vi "Save Controls.vi"(8 "Parent Label":string, 9 "Parent Class":string, 10 "Controls[]":refnum<vi>[](array[refnum]), 11 "Ref Config File In":T1) -> (3 "Ref Config File Out":T1)   [LabVIEW 2009]
uses:
  <vilib>/Utility/config.llb/Config Data RefNum.ctl
  <vilib>/Utility/config.llb/Write Key (Double).vi
  <vilib>/Utility/config.llb/Write Key (Boolean).vi
  <vilib>/Utility/config.llb/Write Key (String).vi
  <vilib>/Utility/config.llb/Write Key (Path).vi
  <vilib>/Utility/config.llb/Write Key (I32).vi
  <vilib>/Utility/config.llb/NI_LVConfig.lvlib
panel:
  # "Guillaume Plateau - Dec. 9, 2009\nyguig2@yahoo.fr - Version 3.0"
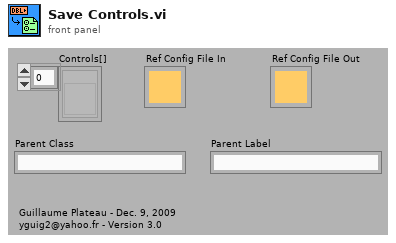
[diagram p1: front panel]
types:
  T1 = typedef "NI_LVConfig.lvlib/Config Data RefNum.ctl" = refnum<k1>
  T2 = enum16{"fractional", "engineering", "exponential"}
  T3 = typedef "LVCursorListTypeDef.ctl" = cluster{"Name":string, "Color":u32, "Style":u8, "Point Style":u8, "Name Visible":bool, "Allow Drag":bool, "Cursor Mode":u32, "Plot":i32, "Index":i32, "Position":cluster{"X":dbl, "Y":dbl}, "X Scale":u32, "Y Scale":u32, "Watch Plots":i32[], "Watch All Plots":bool, "Plot Area":i32, "Label Offset":cluster{"X":dbl, "Y":dbl}}[]
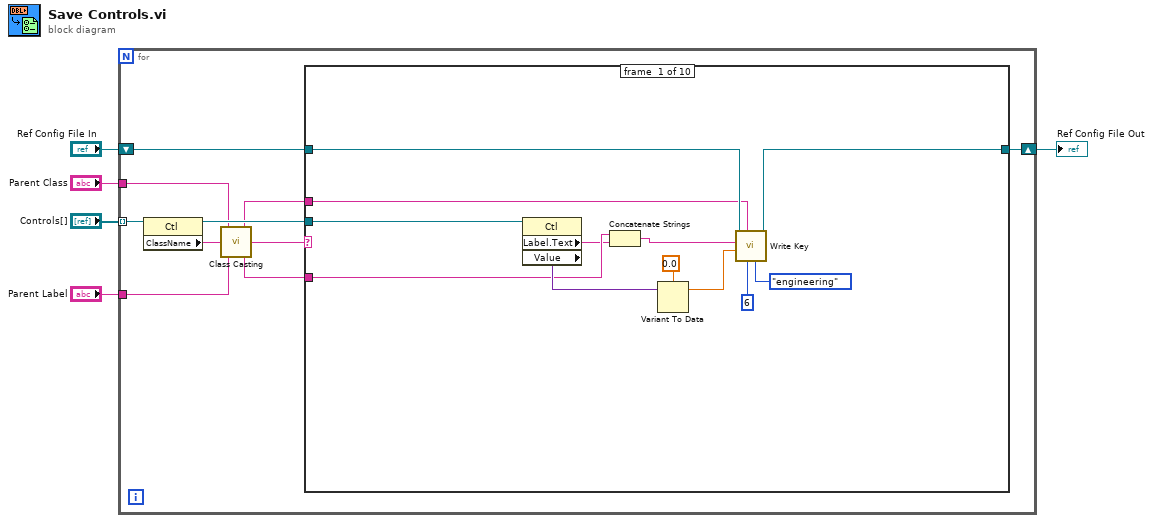
[diagram p0: block diagram]
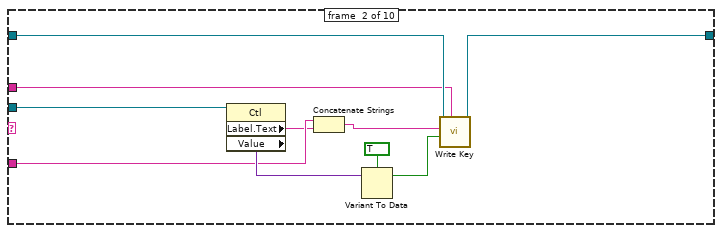
[diagram p2: hidden frame]
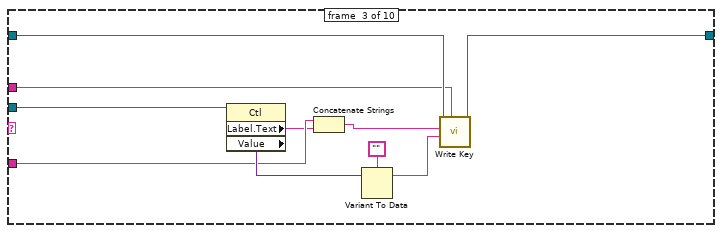
[diagram p3: hidden frame]
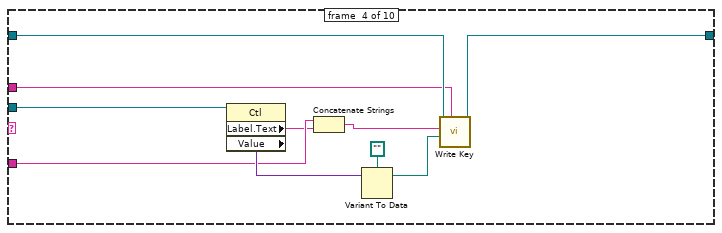
[diagram p4: hidden frame]
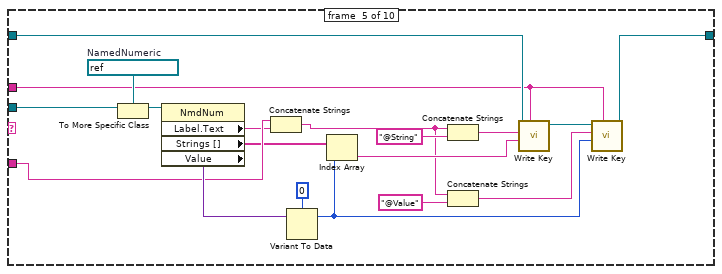
[diagram p5: hidden frame]
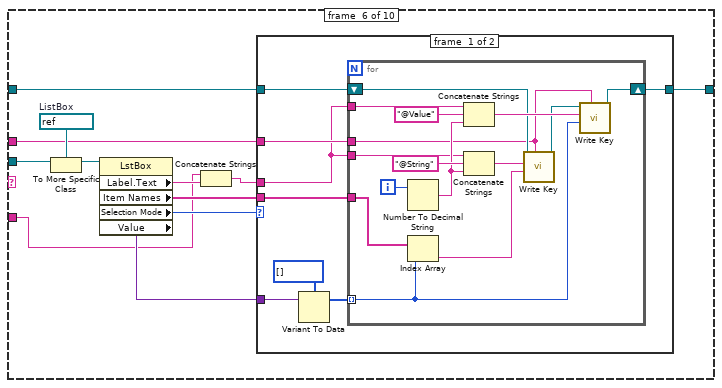
[diagram p6: hidden frame]
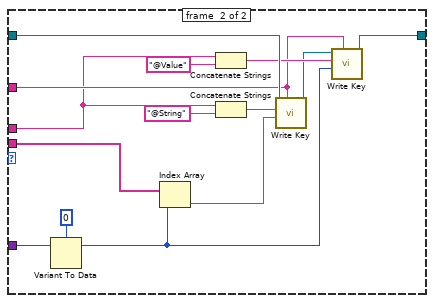
[diagram p7: hidden frame]
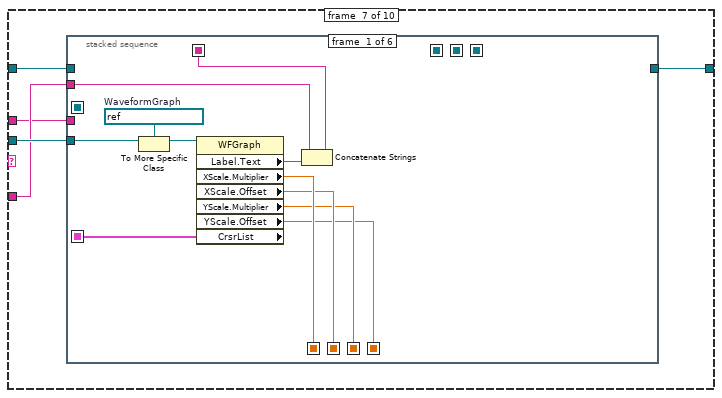
[diagram p8: hidden frame]
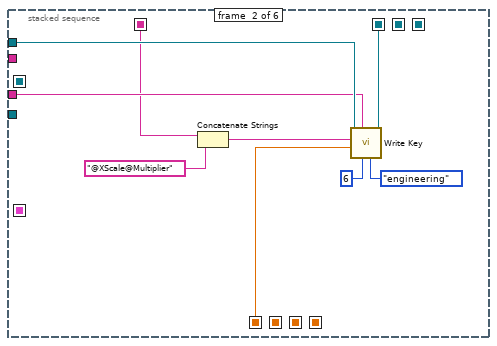
[diagram p9: hidden frame]
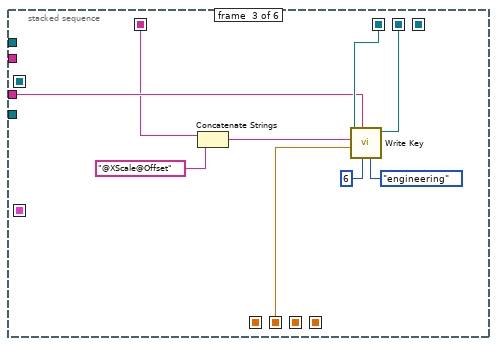
[diagram p10: hidden frame]
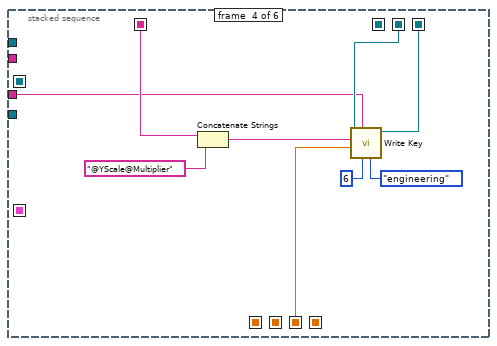
[diagram p11: hidden frame]
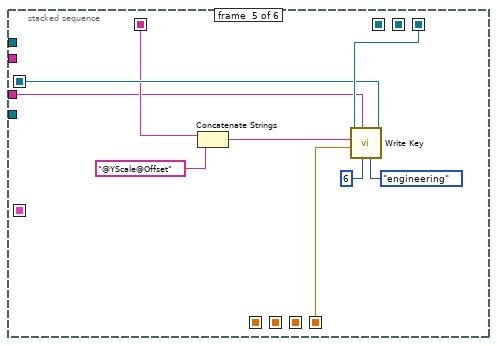
[diagram p12: hidden frame]
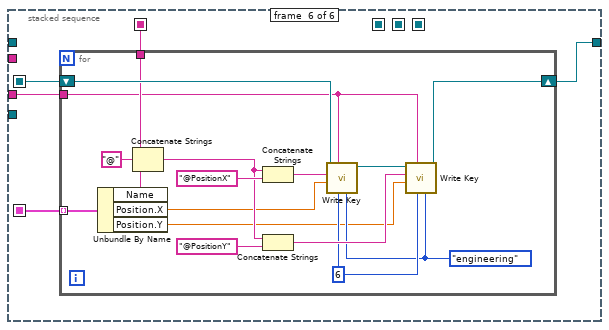
[diagram p13: hidden frame]
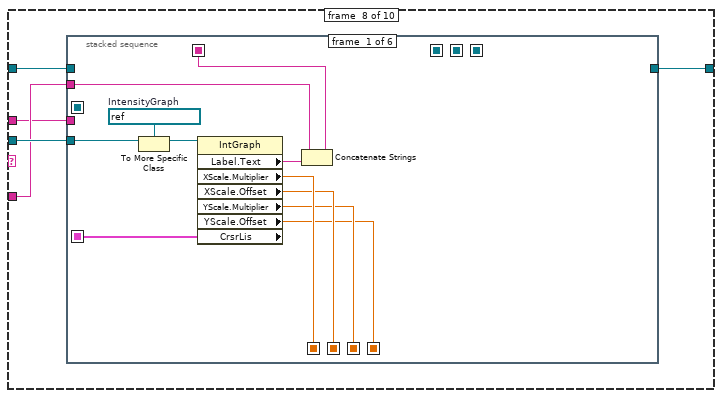
[diagram p14: hidden frame]
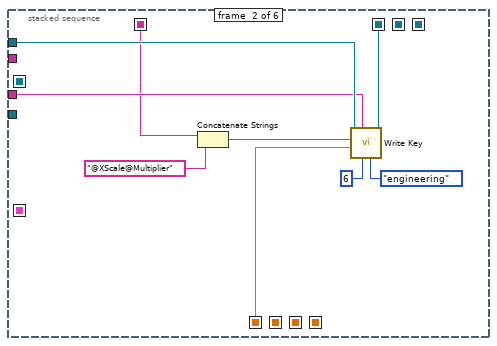
[diagram p15: hidden frame]
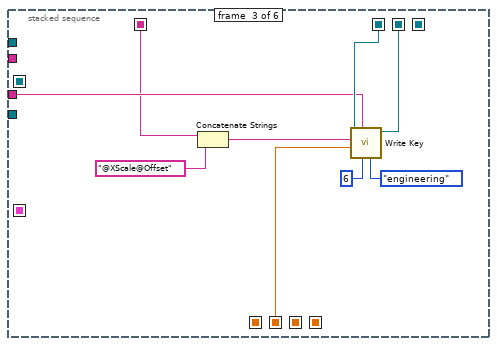
[diagram p16: hidden frame]
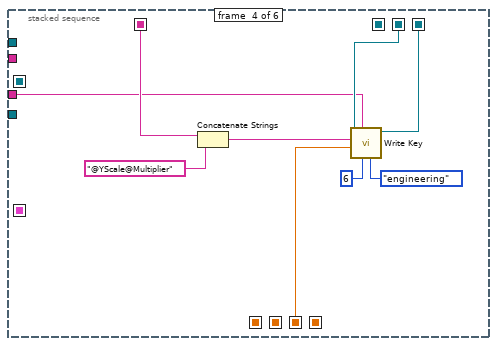
[diagram p17: hidden frame]
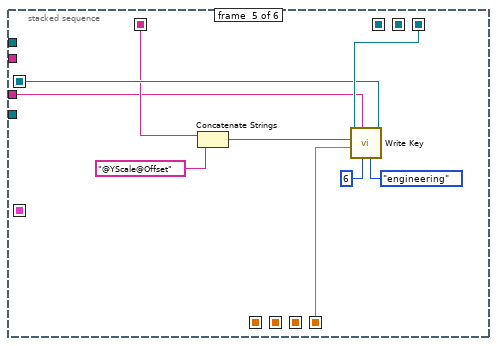
[diagram p18: hidden frame]
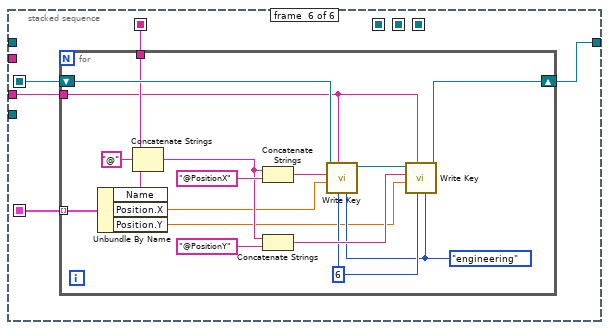
[diagram p19: hidden frame]
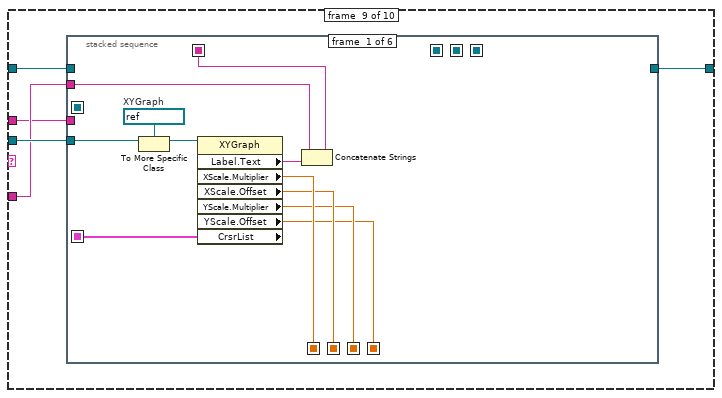
[diagram p20: hidden frame]
diagram:
  n1 = for {
    tunnel: "Controls[]" -> [w12] mode=indexing
    shift-right: [w13] -> w5
    shift-left: "Ref Config File In" -> [w14]
    tunnel: "Parent Class" -> [w7]
    tunnel: "Parent Label" -> [w11]
    n2 = property class="Ctl"(reference=w12) -> (reference out=w9:refnum<vi>, "ClassName"=w8:string)  [unwired: 1 in, 1 out]
    n3 = call "Class Casting.vi"("Parent Label"=w11, "Control Class"=w8, "Parent Class"=w7) -> ("Add-on Label"=w10:string, "Class"=w6:string)  [unwired: 1 out]
    n4 = case shown="\"OtherClasses\", Default" w8 {
      tunnel: w9 -> [w25 w27 w45 w55 w74 w87 w129 w203 w277 _]
      tunnel: w14 -> [w23 w34 w43 w53 w67 w83 w128 w202 w276 w347]
      tunnel: [w20 w32 w41 w52 w75 w80 w127 w201 w275 w347] -> w13
      tunnel: w10 -> [w19 w30 w39 w49 w61 w77 w126 w200 w274 _]
      tunnel: w6 -> [w16 w28 w37 w47 w57 w76 w125 w199 w273 _]
      frame #0 {
        n5 = property class="Ctl"(reference=w25) -> ("Label.Text"=w17:string, "Value"=w24:variant)  [unwired: 1 in, 2 out]
        n6 = Concatenate Strings(w19, w17) -> (w18:string)
        n7 = Variant To Data(Variant=w24, type=0.0) -> (data=w15:dbl)  [unwired: 1 in, 1 out]
        n8 = call-poly <vilib>:"Write Key.vi"("format (fractional)"=T2."engineering", "precision (6)"=i16 6, "section"=w16, "value"=w15, "key"=w18, "refnum"=w23) -> ("refnum out"=w20:T1)  [unwired: 2 in, 3 out]
      }
      frame #1 {
        n9 = property class="Ctl"(reference=w27) -> ("Label.Text"=w29:string, "Value"=w35:variant)  [unwired: 1 in, 2 out]
        n10 = Concatenate Strings(w30, w29) -> (w31:string)
        n11 = Variant To Data(Variant=w35, type=TRUE) -> (data=w33:bool)  [unwired: 1 in, 1 out]
        n12 = call-poly <vilib>:"Write Key.vi"("section"=w28, "value"=w33, "key"=w31, "refnum"=w34) -> ("refnum out"=w32:T1)  [unwired: 3 in, 4 out]
      }
      frame #2 {
        n13 = property class="Ctl"(reference=w45) -> ("Label.Text"=w38:string, "Value"=w44:variant)  [unwired: 1 in, 2 out]
        n14 = Concatenate Strings(w39, w38) -> (w40:string)
        n15 = Variant To Data(Variant=w44, type="") -> (data=w42:string)  [unwired: 1 in, 1 out]
        n16 = call-poly <vilib>:"Write Key.vi"("section"=w37, "value"=w42, "key"=w40, "refnum"=w43) -> ("refnum out"=w41:T1)  [unwired: 3 in, 4 out]
      }
      frame #3 {
        n17 = property class="Ctl"(reference=w55) -> ("Label.Text"=w48:string, "Value"=w54:variant)  [unwired: 1 in, 2 out]
        n18 = Concatenate Strings(w49, w48) -> (w50:string)
        n19 = Variant To Data(Variant=w54, type=path "") -> (data=w51:path)  [unwired: 1 in, 1 out]
        n20 = call-poly <vilib>:"Write Key.vi"("section"=w47, "value"=w51, "key"=w50, "refnum"=w53) -> ("refnum out"=w52:T1)  [unwired: 3 in, 4 out]
      }
      frame #4 {
        w73 = refnum<vi> refnum  # NamedNumeric
        n21 = To More Specific Class(target class=w73, reference=w74) -> (specific class reference=w72:refnum<vi>)  [unwired: 1 in, 1 out]
        n22 = property class="NmdNum"(reference=w72) -> ("Label.Text"=w60:string, "Strings []"=w58:string[], "Value"=w70:variant)  [unwired: 1 in, 2 out]
        n23 = Concatenate Strings(w61, w60) -> (w59:string)
        n24 = Variant To Data(Variant=w70, type=0) -> (data=w63:i32)  [unwired: 1 in, 1 out]
        n25 = Index Array(array=w58, index=w63) -> (element=w62:string)
        n26 = Concatenate Strings(w59, "@String" ("string")) -> (w64:string)
        n27 = Concatenate Strings(w59, "@Value" ("string")) -> (w65:string)
        n28 = call-poly <vilib>:"Write Key.vi"("section"=w57, "value"=w62, "key"=w64, "refnum"=w67) -> ("refnum out"=w66:T1)  [unwired: 2 in, 5 out]
        n29 = call-poly <vilib>:"Write Key.vi"("section"=w57, "value"=w63, "key"=w65, "refnum"=w66) -> ("refnum out"=w75:T1)  [unwired: 1 in, 6 out]
      }
      frame #5 {
        w86 = refnum<vi> refnum  # ListBox
        n30 = To More Specific Class(target class=w86, reference=w87) -> (specific class reference=w85:refnum<vi>)  [unwired: 1 in, 1 out]
        n31 = property class="LstBox"(reference=w85) -> ("Label.Text"=w79:string, "Item Names"=w81:string[], "Selection Mode"=w84:i32, "Value"=w82:variant)  [unwired: 1 in, 2 out]
        n32 = Concatenate Strings(w77, w79) -> (w78:string)
        n33 = case shown="2, 3" w84 {
          tunnel: w83 -> [w94 w124]
          tunnel: w82 -> [w93 w123]
          tunnel: w81 -> [w91 w121]
          tunnel: w76 -> [w90 w113]
          tunnel: w78 -> [w89 w112]
          tunnel: [w88 w111] -> w80
          frame #0 {
            n34 = Variant To Data(Variant=w93, type=i32[] []) -> (data=w92:i32[])  [unwired: 1 in, 1 out]
            n35 = for {
              shift-right: [w102] -> w88
              shift-left: w94 -> [w103]
              tunnel: w92 -> [w100] mode=indexing
              tunnel: w91 -> [w101]
              tunnel: w90 -> [w98]
              tunnel: w89 -> [w97]
              tunnel: w89 -> [w96]
              i -> [w108]
              n36 = Number To Decimal String(number=w108) -> (decimal integer string=w105:string)  [unwired: 1 out]
              n37 = Index Array(array=w101, index=w100) -> (element=w99:string)
              n38 = Concatenate Strings(w96, "@Value" ("string"), w105) -> (w109:string)
              n39 = Concatenate Strings(w97, "@String" ("string"), w105) -> (w107:string)
              n40 = call-poly <vilib>:"Write Key.vi"("section"=w98, "value"=w99, "key"=w107, "refnum"=w103) -> ("refnum out"=w104:T1)  [unwired: 2 in, 5 out]
              n41 = call-poly <vilib>:"Write Key.vi"("section"=w98, "value"=w100, "key"=w109, "refnum"=w104) -> ("refnum out"=w102:T1)  [unwired: 1 in, 6 out]
            }
          }
          frame #1 {
            n42 = Variant To Data(Variant=w123, type=0) -> (data=w122:i32)  [unwired: 1 in, 1 out]
            n43 = Index Array(array=w121, index=w122) -> (element=w114:string)
            n44 = Concatenate Strings(w112, "@Value" ("string")) -> (w118:string)
            n45 = Concatenate Strings(w112, "@String" ("string")) -> (w117:string)
            n46 = call-poly <vilib>:"Write Key.vi"("section"=w113, "value"=w114, "key"=w117, "refnum"=w124) -> ("refnum out"=w115:T1)  [unwired: 2 in, 5 out]
            n47 = call-poly <vilib>:"Write Key.vi"("section"=w113, "value"=w122, "key"=w118, "refnum"=w115) -> ("refnum out"=w111:T1)  [unwired: 1 in, 6 out]
          }
        }
      }
      frame #6 {
        n48 = stacked-sequence {
          seq-local: [w137 _ _ _ _ _] -> [_ _ _ _ _ w181]
          seq-local: [_ _ _ _ w170 _] -> [_ _ _ _ _ w180]
          seq-local: [w136 _ _ _ _ _] -> [_ w147 _ _ _ _]
          seq-local: [w135 _ _ _ _ _] -> [_ _ w152 _ _ _]
          seq-local: [w134 _ _ _ _ _] -> [_ _ _ w161 _ _]
          seq-local: [w133 _ _ _ _ _] -> [_ _ _ _ w171 _]
          seq-local: [_ w143 _ _ _ _] -> [_ _ w154 _ _ _]
          seq-local: [_ _ w153 _ _ _] -> [_ _ _ w163 _ _]
          seq-local: [_ _ _ w162 _ _] -> [_ _ _ _ w172 _]
          seq-local: [w130 _ _ _ _ _] -> [_ w141 w150 w160 w169 w178]
          tunnel: w129 -> [w138 _ _ _ _ _]
          tunnel: w128 -> [_ w144 _ _ _ _]
          tunnel: [_ _ _ _ _ w179] -> w127
          tunnel: w125 -> [_ w142 w151 w159 w168 w177]
          tunnel: w126 -> [w131 _ _ _ _ _]
          frame #0 {
            w140 = refnum<vi> refnum  # WaveformGraph
            n49 = To More Specific Class(target class=w140, reference=w138) -> (specific class reference=w139:refnum<vi>)  [unwired: 1 in, 1 out]
            n50 = property class="WFGraph"(reference=w139) -> ("Label.Text"=w132:string, "XScale.Multiplier"=w136:dbl, "XScale.Offset"=w135:dbl, "YScale.Multiplier"=w134:dbl, "YScale.Offset"=w133:dbl, "CrsrList"=w137:T3)  [unwired: 1 in, 2 out]
            n51 = Concatenate Strings(w131, w132) -> (w130:string)
          }
          frame #1 {
            n52 = Concatenate Strings(w141, "@XScale@Multiplier" ("string")) -> (w145:string)
            n53 = call-poly <vilib>:"Write Key.vi"("format (fractional)"=T2."engineering", "precision (6)"=i16 6, "section"=w142, "value"=w147, "key"=w145, "refnum"=w144) -> ("refnum out"=w143:T1)  [unwired: 2 in, 3 out]
          }
          frame #2 {
            n54 = Concatenate Strings(w150, "@XScale@Offset" ("string")) -> (w155:string)
            n55 = call-poly <vilib>:"Write Key.vi"("format (fractional)"=T2."engineering", "precision (6)"=i16 6, "section"=w151, "value"=w152, "key"=w155, "refnum"=w154) -> ("refnum out"=w153:T1)  [unwired: 2 in, 3 out]
          }
          frame #3 {
            n56 = Concatenate Strings(w160, "@YScale@Multiplier" ("string")) -> (w164:string)
            n57 = call-poly <vilib>:"Write Key.vi"("format (fractional)"=T2."engineering", "precision (6)"=i16 6, "section"=w159, "value"=w161, "key"=w164, "refnum"=w163) -> ("refnum out"=w162:T1)  [unwired: 2 in, 3 out]
          }
          frame #4 {
            n58 = Concatenate Strings(w169, "@YScale@Offset" ("string")) -> (w173:string)
            n59 = call-poly <vilib>:"Write Key.vi"("format (fractional)"=T2."engineering", "precision (6)"=i16 6, "section"=w168, "value"=w171, "key"=w173, "refnum"=w172) -> ("refnum out"=w170:T1)  [unwired: 2 in, 3 out]
          }
          frame #5 {
            n60 = for {
              shift-right: [w186] -> w179
              shift-left: w180 -> [w187]
              tunnel: w181 -> [w198] mode=indexing
              tunnel: w178 -> [w183]
              tunnel: w177 -> [w182]
              w190 = T2."engineering" ("format (fractional)")
              w191 = i16 6 ("precision (6)")
              n61 = Unbundle By Name(w198) -> ("Name"=w196:string, "Position.X"=w185:dbl, "Position.Y"=w184:dbl)
              n62 = Concatenate Strings(w183, "@" ("string"), w196) -> (w188:string)
              n63 = Concatenate Strings(w188, "@PositionX" ("string")) -> (w193:string)
              n64 = Concatenate Strings(w188, "@PositionY" ("string")) -> (w192:string)
              n65 = call-poly <vilib>:"Write Key.vi"("format (fractional)"=w190, "precision (6)"=w191, "section"=w182, "value"=w185, "key"=w193, "refnum"=w187) -> ("refnum out"=w189:T1)  [unwired: 2 in, 3 out]
              n66 = call-poly <vilib>:"Write Key.vi"("format (fractional)"=w190, "precision (6)"=w191, "section"=w182, "value"=w184, "key"=w192, "refnum"=w189) -> ("refnum out"=w186:T1)  [unwired: 2 in, 3 out]
            }
          }
        }
      }
      frame #7 {
        n67 = stacked-sequence {
          seq-local: [w211 _ _ _ _ _] -> [_ _ _ _ _ w255]
          seq-local: [_ _ _ _ w244 _] -> [_ _ _ _ _ w254]
          seq-local: [w210 _ _ _ _ _] -> [_ w221 _ _ _ _]
          seq-local: [w209 _ _ _ _ _] -> [_ _ w226 _ _ _]
          seq-local: [w208 _ _ _ _ _] -> [_ _ _ w235 _ _]
          seq-local: [w207 _ _ _ _ _] -> [_ _ _ _ w245 _]
          seq-local: [_ w217 _ _ _ _] -> [_ _ w228 _ _ _]
          seq-local: [_ _ w227 _ _ _] -> [_ _ _ w237 _ _]
          seq-local: [_ _ _ w236 _ _] -> [_ _ _ _ w246 _]
          seq-local: [w204 _ _ _ _ _] -> [_ w215 w224 w234 w243 w252]
          tunnel: w203 -> [w212 _ _ _ _ _]
          tunnel: w202 -> [_ w218 _ _ _ _]
          tunnel: [_ _ _ _ _ w253] -> w201
          tunnel: w199 -> [_ w216 w225 w233 w242 w251]
          tunnel: w200 -> [w205 _ _ _ _ _]
          frame #0 {
            w214 = refnum<vi> refnum  # IntensityGraph
            n68 = To More Specific Class(target class=w214, reference=w212) -> (specific class reference=w213:refnum<vi>)  [unwired: 1 in, 1 out]
            n69 = property class="IntGraph"(reference=w213) -> ("Label.Text"=w206:string, "XScale.Multiplier"=w210:dbl, "XScale.Offset"=w209:dbl, "YScale.Multiplier"=w208:dbl, "YScale.Offset"=w207:dbl, "CrsrLis"=w211:T3)  [unwired: 1 in, 2 out]
            n70 = Concatenate Strings(w205, w206) -> (w204:string)
          }
          frame #1 {
            n71 = Concatenate Strings(w215, "@XScale@Multiplier" ("string")) -> (w219:string)
            n72 = call-poly <vilib>:"Write Key.vi"("format (fractional)"=T2."engineering", "precision (6)"=i16 6, "section"=w216, "value"=w221, "key"=w219, "refnum"=w218) -> ("refnum out"=w217:T1)  [unwired: 2 in, 3 out]
          }
          frame #2 {
            n73 = Concatenate Strings(w224, "@XScale@Offset" ("string")) -> (w229:string)
            n74 = call-poly <vilib>:"Write Key.vi"("format (fractional)"=T2."engineering", "precision (6)"=i16 6, "section"=w225, "value"=w226, "key"=w229, "refnum"=w228) -> ("refnum out"=w227:T1)  [unwired: 2 in, 3 out]
          }
          frame #3 {
            n75 = Concatenate Strings(w234, "@YScale@Multiplier" ("string")) -> (w238:string)
            n76 = call-poly <vilib>:"Write Key.vi"("format (fractional)"=T2."engineering", "precision (6)"=i16 6, "section"=w233, "value"=w235, "key"=w238, "refnum"=w237) -> ("refnum out"=w236:T1)  [unwired: 2 in, 3 out]
          }
          frame #4 {
            n77 = Concatenate Strings(w243, "@YScale@Offset" ("string")) -> (w247:string)
            n78 = call-poly <vilib>:"Write Key.vi"("format (fractional)"=T2."engineering", "precision (6)"=i16 6, "section"=w242, "value"=w245, "key"=w247, "refnum"=w246) -> ("refnum out"=w244:T1)  [unwired: 2 in, 3 out]
          }
          frame #5 {
            n79 = for {
              shift-right: [w260] -> w253
              shift-left: w254 -> [w261]
              tunnel: w255 -> [w272] mode=indexing
              tunnel: w252 -> [w257]
              tunnel: w251 -> [w256]
              w264 = T2."engineering" ("format (fractional)")
              w265 = i16 6 ("precision (6)")
              n80 = Unbundle By Name(w272) -> ("Name"=w270:string, "Position.X"=w259:dbl, "Position.Y"=w258:dbl)
              n81 = Concatenate Strings(w257, "@" ("string"), w270) -> (w262:string)
              n82 = Concatenate Strings(w262, "@PositionX" ("string")) -> (w267:string)
              n83 = Concatenate Strings(w262, "@PositionY" ("string")) -> (w266:string)
              n84 = call-poly <vilib>:"Write Key.vi"("format (fractional)"=w264, "precision (6)"=w265, "section"=w256, "value"=w259, "key"=w267, "refnum"=w261) -> ("refnum out"=w263:T1)  [unwired: 2 in, 3 out]
              n85 = call-poly <vilib>:"Write Key.vi"("format (fractional)"=w264, "precision (6)"=w265, "section"=w256, "value"=w258, "key"=w266, "refnum"=w263) -> ("refnum out"=w260:T1)  [unwired: 2 in, 3 out]
            }
          }
        }
      }
      frame #8 {
        n86 = stacked-sequence {
          seq-local: [w285 _ _ _ _ _] -> [_ _ _ _ _ w329]
          seq-local: [_ _ _ _ w318 _] -> [_ _ _ _ _ w328]
          seq-local: [w284 _ _ _ _ _] -> [_ w295 _ _ _ _]
          seq-local: [w283 _ _ _ _ _] -> [_ _ w300 _ _ _]
          seq-local: [w282 _ _ _ _ _] -> [_ _ _ w309 _ _]
          seq-local: [w281 _ _ _ _ _] -> [_ _ _ _ w319 _]
          seq-local: [_ w291 _ _ _ _] -> [_ _ w302 _ _ _]
          seq-local: [_ _ w301 _ _ _] -> [_ _ _ w311 _ _]
          seq-local: [_ _ _ w310 _ _] -> [_ _ _ _ w320 _]
          seq-local: [w278 _ _ _ _ _] -> [_ w289 w298 w308 w317 w326]
          tunnel: w277 -> [w286 _ _ _ _ _]
          tunnel: w276 -> [_ w292 _ _ _ _]
          tunnel: [_ _ _ _ _ w327] -> w275
          tunnel: w273 -> [_ w290 w299 w307 w316 w325]
          tunnel: w274 -> [w279 _ _ _ _ _]
          frame #0 {
            w288 = refnum<vi> refnum  # XYGraph
            n87 = To More Specific Class(target class=w288, reference=w286) -> (specific class reference=w287:refnum<vi>)  [unwired: 1 in, 1 out]
            n88 = property class="XYGraph"(reference=w287) -> ("Label.Text"=w280:string, "XScale.Multiplier"=w284:dbl, "XScale.Offset"=w283:dbl, "YScale.Multiplier"=w282:dbl, "YScale.Offset"=w281:dbl, "CrsrList"=w285:T3)  [unwired: 1 in, 2 out]
            n89 = Concatenate Strings(w279, w280) -> (w278:string)
          }
          frame #1 {
            n90 = Concatenate Strings(w289, "@XScale@Multiplier" ("string")) -> (w293:string)
            n91 = call-poly <vilib>:"Write Key.vi"("format (fractional)"=T2."engineering", "precision (6)"=i16 6, "section"=w290, "value"=w295, "key"=w293, "refnum"=w292) -> ("refnum out"=w291:T1)  [unwired: 2 in, 3 out]
          }
          frame #2 {
            n92 = Concatenate Strings(w298, "@XScale@Offset" ("string")) -> (w303:string)
            n93 = call-poly <vilib>:"Write Key.vi"("format (fractional)"=T2."engineering", "precision (6)"=i16 6, "section"=w299, "value"=w300, "key"=w303, "refnum"=w302) -> ("refnum out"=w301:T1)  [unwired: 2 in, 3 out]
          }
          frame #3 {
            n94 = Concatenate Strings(w308, "@YScale@Multiplier" ("string")) -> (w312:string)
            n95 = call-poly <vilib>:"Write Key.vi"("format (fractional)"=T2."engineering", "precision (6)"=i16 6, "section"=w307, "value"=w309, "key"=w312, "refnum"=w311) -> ("refnum out"=w310:T1)  [unwired: 2 in, 3 out]
          }
          frame #4 {
            n96 = Concatenate Strings(w317, "@YScale@Offset" ("string")) -> (w321:string)
            n97 = call-poly <vilib>:"Write Key.vi"("format (fractional)"=T2."engineering", "precision (6)"=i16 6, "section"=w316, "value"=w319, "key"=w321, "refnum"=w320) -> ("refnum out"=w318:T1)  [unwired: 2 in, 3 out]
          }
          frame #5 {
            n98 = for {
              shift-right: [w334] -> w327
              shift-left: w328 -> [w335]
              tunnel: w329 -> [w346] mode=indexing
              tunnel: w326 -> [w331]
              tunnel: w325 -> [w330]
              w338 = T2."engineering" ("format (fractional)")
              w339 = i16 6 ("precision (6)")
              n99 = Unbundle By Name(w346) -> ("Name"=w344:string, "Position.X"=w333:dbl, "Position.Y"=w332:dbl)
              n100 = Concatenate Strings(w331, "@" ("string"), w344) -> (w336:string)
              n101 = Concatenate Strings(w336, "@PositionX" ("string")) -> (w341:string)
              n102 = Concatenate Strings(w336, "@PositionY" ("string")) -> (w340:string)
              n103 = call-poly <vilib>:"Write Key.vi"("format (fractional)"=w338, "precision (6)"=w339, "section"=w330, "value"=w333, "key"=w341, "refnum"=w335) -> ("refnum out"=w337:T1)  [unwired: 2 in, 3 out]
              n104 = call-poly <vilib>:"Write Key.vi"("format (fractional)"=w338, "precision (6)"=w339, "section"=w330, "value"=w332, "key"=w340, "refnum"=w337) -> ("refnum out"=w334:T1)  [unwired: 2 in, 3 out]
            }
          }
        }
      }
      frame #9 {
      }
    }
  }
  "Ref Config File Out" <- w5
